vi "DemoDataIntesityGraphs.vi"() -> (2 "Array 2":dbl[][](array[numeric]), 3 "Array":dbl[][](array[numeric]), 4 "y offset":dbl, 5 "x offset":dbl, 6 "Y multi":dbl, 7 "x multi":dbl)   [LabVIEW 2022 SP3]
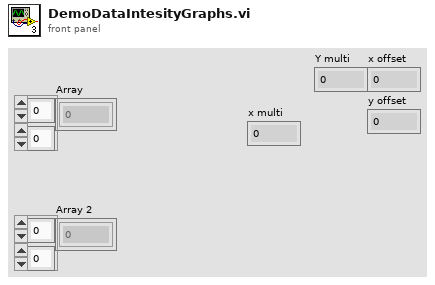
[diagram p1: front panel]
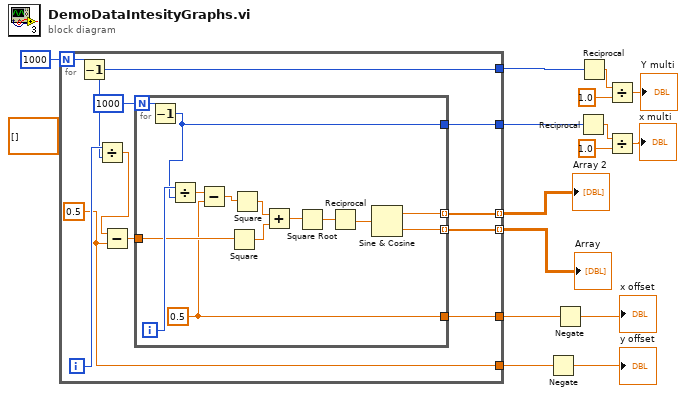
[diagram p0: block diagram]
diagram:
  (unwired) dbl[][] [] ("Intensity Graph")
  n1 = for {
    N: 1000 -> [w26]
    tunnel: [w22] -> w13 mode=indexing
    tunnel: [w21] -> w14 mode=indexing
    tunnel: [w19] -> w10
    tunnel: [w18] -> w8
    tunnel: [w17] -> w4
    tunnel: [w16] -> w2
    i -> [w25]
    w18 = 0.5 ("y")
    n2 = Decrement(x=w26) -> (x-1=w17:i32)
    n3 = Divide(x=w25, y=w17) -> (x/y=w24:dbl)
    n4 = Subtract(x=w24, y=w18) -> (x-y=w23:dbl)
    n5 = for {
      N: 1000 -> [w39]
      tunnel: w23 -> [w36]
      tunnel: [w30] -> w22 mode=indexing
      tunnel: [w29] -> w21 mode=indexing
      tunnel: [w28] -> w19
      tunnel: [w27] -> w16
      i -> [w40]
      w27 = 0.5 ("y")
      n6 = Decrement(x=w39) -> (x-1=w28:i32)
      n7 = Divide(x=w40, y=w28) -> (x/y=w38:dbl)
      n8 = Subtract(x=w38, y=w27) -> (x-y=w37:dbl)
      n9 = Square(x=w36) -> (x^2=w35:dbl)
      n10 = Square(x=w37) -> (x^2=w34:dbl)
      n11 = Add(x=w34, y=w35) -> (x+y=w33:dbl)
      n12 = Square Root(x=w33) -> (sqrt(x)=w32:dbl)
      n13 = Reciprocal(x=w32) -> (1/x=w31:dbl)
      n14 = Sine & Cosine(0:w31) -> (1:w30:dbl, 2:w29:dbl)
    }
  }
  "Array" <- w14
  "Array 2" <- w13
  n15 = Negate(x=w8) -> (-x=→"y offset":dbl)
  n16 = Negate(x=w2) -> (-x=→"x offset":dbl)
  n17 = Reciprocal(x=w10) -> (1/x=w12:dbl)
  n18 = Reciprocal(x=w4) -> (1/x=w6:dbl)
  n19 = Divide(x=w6, y=1.0) -> (x/y=→"Y multi":dbl)
  n20 = Divide(x=w12, y=1.0) -> (x/y=→"x multi":dbl)
